vi "DCVoltage.vi"() -> ()   [LabVIEW 2014]
uses:
  <vilib>/Utility/error.llb/DialogType.ctl
  <vilib>/DAQmx/write.llb/DAQmx Write (Analog 1D Wfm NChan NSamp).vi
  <vilib>/DAQmx/create/channels.llb/DAQmx Create Channel (AO-Voltage-Basic).vi
  <vilib>/DAQmx/configure/timing.llb/DAQmx Timing (Sample Clock).vi
  <vilib>/DAQmx/miscellaneous.llb/DAQmx Fill In Error Info.vi
  <resource>/objmgr/daqmx.rc
panel:
  in  "SCAN":bool
  out "Z 2":dbl
  in  "interval_z":dbl=0.5
  in  "interval_y":dbl=0.5
  out "Y 2":dbl
  out "X 2":dbl
  in  "interval_x":dbl=0.5
  in  "Increase":bool
  in  "Z":dbl=2.1 caption="Offset"
  in  "Reset":bool
  in  "samples per channel":i32=12101
  in  "Y":dbl=5.55 caption="Offset"
  in  "X":dbl=3.35 caption="Offset"
  in  "Sample Rate":dbl=1000000.0
  in  "Sample Clock Source":tag="OnboardClock"
  in  "Max Voltage":dbl=10.0
  in  "Min Voltage":dbl=-10.0
  in  "Physical Channel(s)":tag="Dev1/ao0,Dev1/ao1,Dev1/ao3"
  out "Actual Sample Rate":dbl=1000.0 format="%0.2f"
  in  "Stop":bool
  out "Waveform Graph":dynamicdata(graph)
  # "5e4 = 1s"
  # "3.35"
  # "X"
  # "Y"
  # "5.55"
  # "2.1"
  # "y = 125"
  # "1.060958"
  # "3.139042"
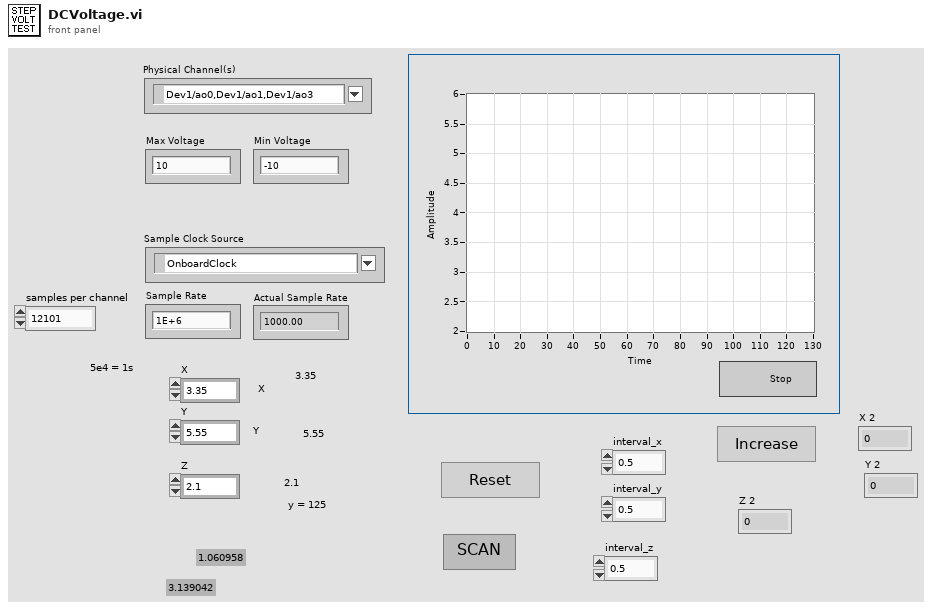
[diagram p1: front panel]
types:
  T1 = typedef "DialogType.ctl" = u16
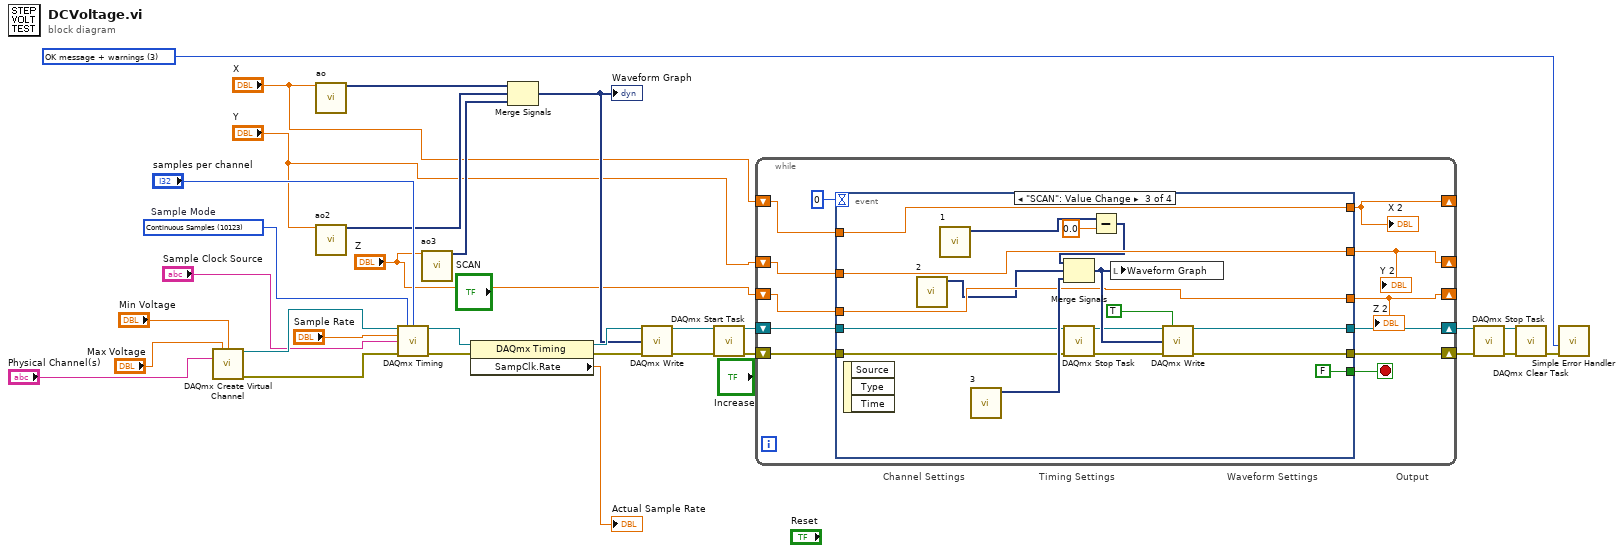
[diagram p0: block diagram]
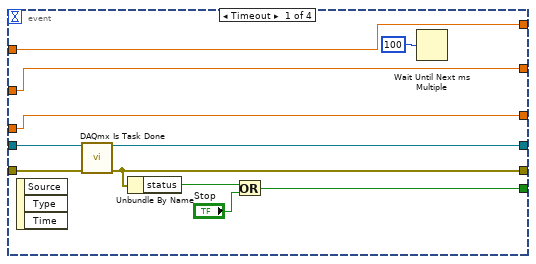
[diagram p2: hidden frame]
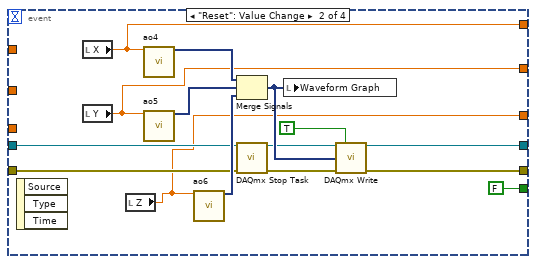
[diagram p3: hidden frame]
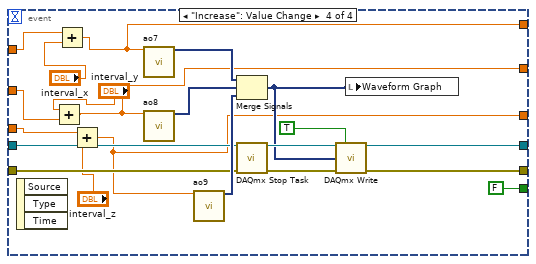
[diagram p4: hidden frame]
diagram:
  w13 = T1 3 items=["no dialog", "OK message", "continue or stop message", "OK message + warnings", "continue/stop + warnings"] ("type of dialog (OK msg:1)")
  w29 = 10123 items=["Finite Samples"=10178, "Continuous Samples"=10123, "Hardware Timed Single Point"=12522]  # Sample Mode
  # "Output"
  # "Waveform Settings"
  # "Timing Settings"
  # "Channel Settings"
  n1 = call-poly <vilib>:"DAQmx Create Virtual Channel.vi"("maximum value"="Max Voltage", "minimum value"="Min Voltage", "physical channels"="Physical Channel(s)") -> ("task out"=w27:refnum<k21>, "error out"=w28:errorcluster)  [unwired: 11 in]
  n2 = call "ao"("Offset"="X") -> ("DC"=w7:dynamicdata)  [unwired: 13 in, 1 out]
  n3 = call "ao2"("Offset"="Y") -> ("DC"=w6:dynamicdata)  [unwired: 13 in, 1 out]
  n4 = call-poly <vilib>:"DAQmx Timing.vi"("task/channels in"=w27, "sample mode"=w29, "samples per channel"="samples per channel", "rate"="Sample Rate", "source"="Sample Clock Source", "error in"=w28) -> ("task out"=w31:refnum<k21>, "error out"=w30:errorcluster)  [unwired: 8 in]
  n5 = call "ao3"("Offset"="Z") -> ("DC"=w9:dynamicdata)  [unwired: 13 in, 1 out]
  n6 = property class="DAQmx Timing"(reference=w31, error in=w30) -> (reference out=w12:refnum<k21>, error out=w11:errorcluster, "SampClk.Rate"=→"Actual Sample Rate":dbl)
  n7 = Merge Signals(w7, w6, w9) -> (w10:dynamicdata)
  "Waveform Graph" <- w10
  n8 = call-poly <vilib>:"DAQmx Write.vi"("task/channels in"=w12, "data"=w10, "error in"=w11) -> ("task out"=w17:refnum<k21>, "error out"=w16:errorcluster)  [unwired: 10 in, 1 out]
  n9 = call <vilib>:"DAQmx Start Task.vi"("task/channels in"=w17, "error in"=w16) -> ("task out"=w26:refnum<k21>, "error out"=w25:errorcluster)  [unwired: 12 in]
  n10 = while {
    shift-right: [w40] -> w5
    shift-left: w26 -> [w42]
    shift-right: [w39] -> w4
    shift-left: w25 -> [w41]
    shift-right: [w35] -> _
    shift-left: "X" -> [w37]
    shift-right: [w34] -> _
    shift-left: "Y" -> [w36]
    shift-right: [w32] -> _
    shift-left: "Z" -> [w33]
    stop <- w43 stop-if-true
    n11 = event shown="[2] \"SCAN\": Value Change" {
      selector: _ -> [_ _ _ _]
      dyn-events: _ -> [_ _ _ _]
      timeout: 0 -> [_ _ _ _]
      tunnel: [w51 FALSE FALSE FALSE] -> w43
      tunnel: w42 -> [w50 w61 w80 w100]
      tunnel: w41 -> [w49 w60 w79 w99]
      tunnel: [w48 w63 w82 w102] -> w40
      tunnel: [w47 w62 w81 w101] -> w39
      tunnel: w37 -> [w46 _ w75 w94]
      tunnel: w36 -> [w45 _ w74 w92]
      tunnel: [w46 w57 w75 w93] -> w35
      tunnel: [w45 w56 w74 w91] -> w34
      tunnel: w33 -> [w44 _ w76 w89]
      tunnel: [w44 w55 w76 w87] -> w32
      event Timeout {
        n12 = event-data() -> ()  [unwired: 1 in, 3 out]
        n13 = call <vilib>:"DAQmx Is Task Done.vi"("task/channels in"=w50, "error in"=w49) -> ("task out"=w48:refnum<k21>, "error out"=w47:errorcluster)  [unwired: 11 in, 1 out]
        n14 = Unbundle By Name(w47) -> ("status"=w52:bool)
        n15 = Or(x=w52, y="Stop") -> (x .or. y?=w51:bool)
        n16 = Wait Until Next ms Multiple(millisecond multiple=u32 100) -> ()  [unwired: 1 out]
      }
      event "Reset": Value Change {
        n17 = event-data() -> ()  [unwired: 1 in, 3 out]
        n18 = local read "X"() -> (w57:dbl)
        n19 = local read "Y"() -> (w56:dbl)
        n20 = local read "Z"() -> (w55:dbl)
        n21 = call "ao4"("Offset"=w57) -> ("DC"=w69:dynamicdata)  [unwired: 13 in, 1 out]
        n22 = call "ao5"("Offset"=w56) -> ("DC"=w68:dynamicdata)  [unwired: 13 in, 1 out]
        n23 = call "ao6"("Offset"=w55) -> ("DC"=w67:dynamicdata)  [unwired: 13 in, 1 out]
        n24 = Merge Signals(w69, w68, w67) -> (w65:dynamicdata)
        n25 = call <vilib>:"DAQmx Stop Task.vi"("task/channels in"=w61, "error in"=w60) -> ("task out"=w59:refnum<k21>, "error out"=w58:errorcluster)  [unwired: 12 in]
        n26 = local write "Waveform Graph"(w65) -> ()
        n27 = call-poly <vilib>:"DAQmx Write.vi"("task/channels in"=w59, "auto start"=TRUE, "data"=w65, "error in"=w58) -> ("task out"=w63:refnum<k21>, "error out"=w62:errorcluster)  [unwired: 9 in, 1 out]
      }
      event "SCAN": Value Change {
        n28 = event-data() -> ()  [unwired: 1 in, 3 out]
        n29 = call "2"() -> ("Signal"=w73:dynamicdata)  [unwired: 9 in, 2 out]
        n30 = call "1"() -> ("Signal"=w72:dynamicdata)  [unwired: 9 in, 2 out]
        n31 = call "3"() -> ("Signal"=w86:dynamicdata)  [unwired: 9 in, 2 out]
        n32 = call <vilib>:"DAQmx Stop Task.vi"("task/channels in"=w80, "error in"=w79) -> ("task out"=w78:refnum<k21>, "error out"=w77:errorcluster)  [unwired: 12 in]
        n33 = Subtract(x=w72, y=0.0) -> (x-y=w70:dynamicdata)
        n34 = Merge Signals(w70, w73, w86) -> (w84:dynamicdata)
        n35 = local write "Waveform Graph"(w84) -> ()
        n36 = call-poly <vilib>:"DAQmx Write.vi"("task/channels in"=w78, "auto start"=TRUE, "data"=w84, "error in"=w77) -> ("task out"=w82:refnum<k21>, "error out"=w81:errorcluster)  [unwired: 9 in, 1 out]
      }
      event "Increase": Value Change {
        n37 = event-data() -> ()  [unwired: 1 in, 3 out]
        n38 = Add(x="interval_y", y=w92) -> (x+y=w91:dbl)
        n39 = Add(x=w94, y="interval_x") -> (x+y=w93:dbl)
        n40 = Add(x=w89, y="interval_z") -> (x+y=w87:dbl)
        n41 = call "ao7"("Offset"=w93) -> ("DC"=w107:dynamicdata)  [unwired: 13 in, 1 out]
        n42 = call "ao8"("Offset"=w91) -> ("DC"=w106:dynamicdata)  [unwired: 13 in, 1 out]
        n43 = call "ao9"("Offset"=w87) -> ("DC"=w105:dynamicdata)  [unwired: 13 in, 1 out]
        n44 = Merge Signals(w107, w106, w105) -> (w96:dynamicdata)
        n45 = call <vilib>:"DAQmx Stop Task.vi"("task/channels in"=w100, "error in"=w99) -> ("task out"=w98:refnum<k21>, "error out"=w97:errorcluster)  [unwired: 12 in]
        n46 = call-poly <vilib>:"DAQmx Write.vi"("task/channels in"=w98, "auto start"=TRUE, "data"=w96, "error in"=w97) -> ("task out"=w102:refnum<k21>, "error out"=w101:errorcluster)  [unwired: 9 in, 1 out]
        n47 = local write "Waveform Graph"(w96) -> ()
      }
    }
    "X 2" <- w35
    "Y 2" <- w34
    "Z 2" <- w32
  }
  n48 = call <vilib>:"DAQmx Stop Task.vi"("task/channels in"=w5, "error in"=w4) -> ("task out"=w15:refnum<k21>, "error out"=w14:errorcluster)  [unwired: 12 in]
  n49 = call <vilib>:"DAQmx Clear Task.vi"("task in"=w15, "error in"=w14) -> ("error out"=w24:errorcluster)  [unwired: 13 in]
  n50 = call <vilib>:"Simple Error Handler.vi"("type of dialog (OK msg:1)"=w13, "error in (no error)"=w24) -> ()  [unwired: 3 in, 5 out]
